vi "Teleop.vi"(9 "error in":errorcluster) -> (1 "error out":errorcluster)   [LabVIEW 2017]
doc: "This VI is called for each TeleOp packet received from the DS where the robot is not disabled. It is often used to read from the joysticks and update I/O or to update setpoints for timed control loops. It should complete and return within 20 milliseconds or it may miss DS packets."
uses:
  <vilib>/Platform/TimedLoop/XDataNode/timing_clust.ctl
  <vilib>/Platform/TimedLoop/XDataNode/nitl_modes.ctl
  <vilib>/Platform/TimedLoop/XDataNode/wakeup.ctl
  <vilib>/Rock Robotics/WPI/Utilities/WPI_GetSetVariantRefNum.vi
  <vilib>/platform/TimedLoop/XDataNode/XDataNode.xnode
  <vilib>/Platform/TimedLoop/XDataNode/XDNodeRunTimeDep.lvlib
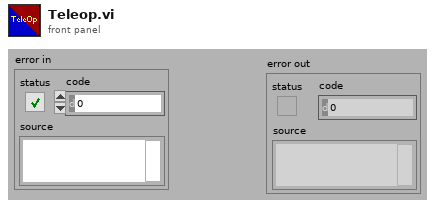
[diagram p1: front panel]
types:
  T1 = typedef "XDNodeRunTimeDep.lvlib/timing_clust.ctl" = cluster{"Expected End [f-1]":u64, "Actual End [f-1]":u64, "Finished Late? [f-1]":bool, "Expected End [i-1]":u64, "Actual End [i-1]":u64, "Finished Late? [i-1]":bool, "Expected Start [i]":u64, "Actual Start [i]":u64, "Expected Start [f]":u64, "Actual Start [f]":u64, "Source Name":string, "Structure Name":string, "Period":i64, "Deadline":i64, "Offset":i64, "Start":i64, "Priority":i32, "Timeout":i32, "Mode":T2, "Wakeup Reason":T3, "Error":errorcluster, "Source Type":string, "Secondary Source Type":string, "Global End Time":u64, "Global Start Time":u64, "Frame Duration":u64, "Iteration Duration":u64, "Assigned CPU":i32, "I/O Scan Engine Mode":u32}
  T2 = typedef "XDNodeRunTimeDep.lvlib/nitl_modes.ctl" = enum32{"No Change", "Process missed periods, maintain original phase", "Discard missed periods, maintain original phase", "Process missed periods, ignore original phase", "Discard missed periods, ignore original phase"}
  T3 = typedef "XDNodeRunTimeDep.lvlib/wakeup.ctl" = enum32{"Normal", "Aborted", "Asynchronous wakeup", "Timing source error", "Timed loop error", "Timeout"}
  T4 = typedef "WPI_JoystickDevRef.ctl" = cluster{"Device":T5}
  T5 = typedef "WPI_JoystickDeviceEnum.ctl" = enum16{"USB 0", "USB 1", "USB 2", "USB 3", "USB 4", "USB 5"}
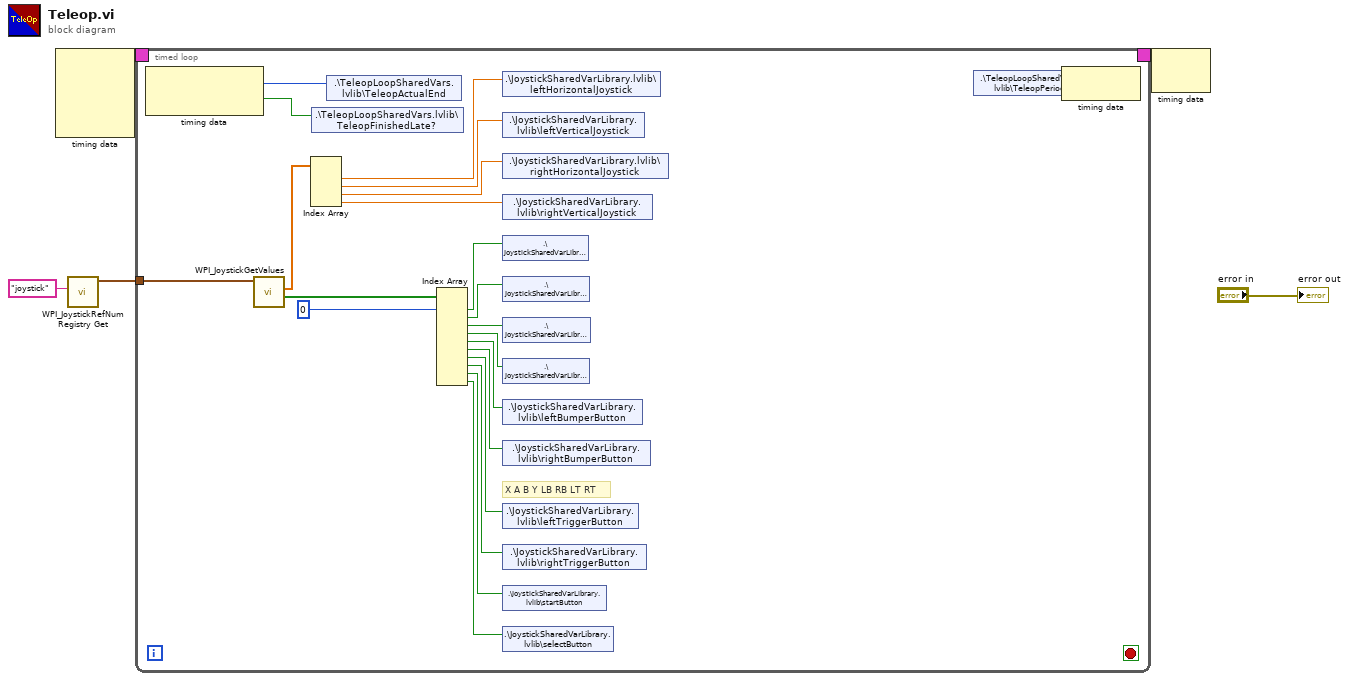
[diagram p0: block diagram]
diagram:
  n1 = node-c288() -> (w5:T1)  [unwired: 4 in]
  n2 = call <vilib>:"WPI_JoystickRefNum Registry Get.vi"("refnum name"="joystick") -> ("JoystickDevRef"=w2:T4)  [unwired: 9 in, 1 out]
  n3 = timed-loop {
    timing: w5 -> [_]
    timing-out: [_] -> w4
    tunnel: w2 -> [w9]
    stop <- _ stop-if-true
    # "X A B Y LB RB LT RT"
    n4 = node-c288() -> (w8:i64, w7:bool)  [unwired: 1 in]
    n5 = call <vilib>:"WPI_JoystickGetValues.vi"("JoystickDevRef"=w9) -> ("Buttons"=w26:bool[], "Axes"=w14:dbl[])  [unwired: 6 in, 3 out]
    n6 = Index Array(array=w14) -> (element #1=w13:dbl, element #2=w12:dbl, element #3=w11:dbl, element #4=w10:dbl)  [unwired: 4 in]
    n7 = shared-variable ".\\TeleopLoopSharedVars.lvlib\\TeleopFinishedLate?"(w7) -> ()  [unwired: 1 in, 1 out]
    n8 = shared-variable ".\\TeleopLoopSharedVars.lvlib\\TeleopActualEnd"(w8) -> ()  [unwired: 1 in, 1 out]
    n9 = Index Array(array=w26, index #1=0) -> (element #1=w24:bool, element #2=w23:bool, element #3=w22:bool, element #4=w21:bool, element #5=w20:bool, element #6=w19:bool, element #7=w18:bool, element #8=w17:bool, element #9=w16:bool, element #10=w15:bool)  [unwired: 9 in]
    n10 = shared-variable ".\\JoystickSharedVarLibrary.lvlib\\leftHorizontalJoystick"(w13) -> ()  [unwired: 1 in, 1 out]
    n11 = shared-variable ".\\JoystickSharedVarLibrary.lvlib\\leftVerticalJoystick"(w12) -> ()  [unwired: 1 in, 1 out]
    n12 = shared-variable ".\\JoystickSharedVarLibrary.lvlib\\rightHorizontalJoystick"(w11) -> ()  [unwired: 1 in, 1 out]
    n13 = shared-variable ".\\JoystickSharedVarLibrary.lvlib\\rightVerticalJoystick"(w10) -> ()  [unwired: 1 in, 1 out]
    n14 = shared-variable ".\\JoystickSharedVarLibrary.lvlib\\xButton"(w24) -> ()  [unwired: 1 in, 1 out]
    n15 = shared-variable ".\\JoystickSharedVarLibrary.lvlib\\aButton"(w23) -> ()  [unwired: 1 in, 1 out]
    n16 = shared-variable ".\\JoystickSharedVarLibrary.lvlib\\bButton"(w22) -> ()  [unwired: 1 in, 1 out]
    n17 = shared-variable ".\\JoystickSharedVarLibrary.lvlib\\yButton"(w21) -> ()  [unwired: 1 in, 1 out]
    n18 = shared-variable ".\\JoystickSharedVarLibrary.lvlib\\leftBumperButton"(w20) -> ()  [unwired: 1 in, 1 out]
    n19 = shared-variable ".\\JoystickSharedVarLibrary.lvlib\\rightBumperButton"(w19) -> ()  [unwired: 1 in, 1 out]
    n20 = shared-variable ".\\JoystickSharedVarLibrary.lvlib\\leftTriggerButton"(w18) -> ()  [unwired: 1 in, 1 out]
    n21 = shared-variable ".\\JoystickSharedVarLibrary.lvlib\\rightTriggerButton"(w17) -> ()  [unwired: 1 in, 1 out]
    n22 = shared-variable ".\\JoystickSharedVarLibrary.lvlib\\startButton"(w16) -> ()  [unwired: 1 in, 1 out]
    n23 = shared-variable ".\\JoystickSharedVarLibrary.lvlib\\selectButton"(w15) -> ()  [unwired: 1 in, 1 out]
    n24 = shared-variable ".\\TeleopLoopSharedVars.lvlib\\TeleopPeriod"() -> (w6:i64)  [unwired: 1 in, 1 out]
    n25 = node-c288(w6) -> ()  [unwired: 1 out]
  }
  n26 = node-c288(w4) -> ()  [unwired: 1 out]
  "error out" <- "error in"
